vi "getStatus.vi"(8 "error in (no error)":errorcluster, 11 "AlCS in":refnum<class "AlCS.lvclass">) -> (0 "error out":errorcluster, 2 "answer":string, 3 "AlCS out":refnum<class "AlCS.lvclass">)   [LabVIEW 2016]
uses:
  AlCS.lvclass
  Parser/CommandCreator.lvclass
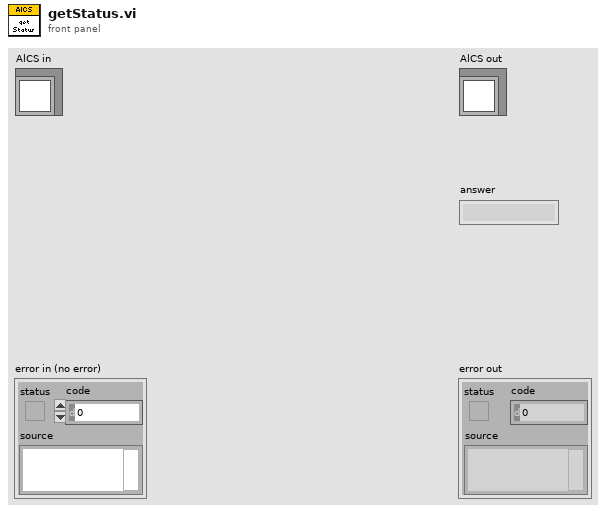
[diagram p1: front panel]
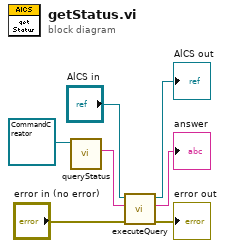
[diagram p0: block diagram]
diagram:
  n1 = call "queryStatus.vi"("CommandCreator in"=refnum<class "CommandCreator.lvclass"> refnum) -> ("command"=w1:string)  [unwired: 8 in, 2 out]
  n2 = call "executeQuery.vi"("error in (no error)"="error in (no error)", "command"=w1, "AlCS in"="AlCS in") -> ("error out"=→"error out":errorcluster, "answer"=→"answer":string, "AlCS out"=→"AlCS out":refnum<class "AlCS.lvclass">)  [unwired: 6 in]
